vi "Put Multiple Files.vi"(3 "remote port (21)":u16=21, 4 "active (T)":bool=TRUE, 5 "password":string, 7 "user":string="anonymous", 8 "error in (no error)":errorcluster, 9 "Open Connection Timeout (ms)":dbl=5000.0, 10 "file specifications":T1(array[cluster]), 11 "host":string) -> (0 "error out":errorcluster, 2 "file errors":errorcluster[](array[cluster]))   [LabVIEW 2023]
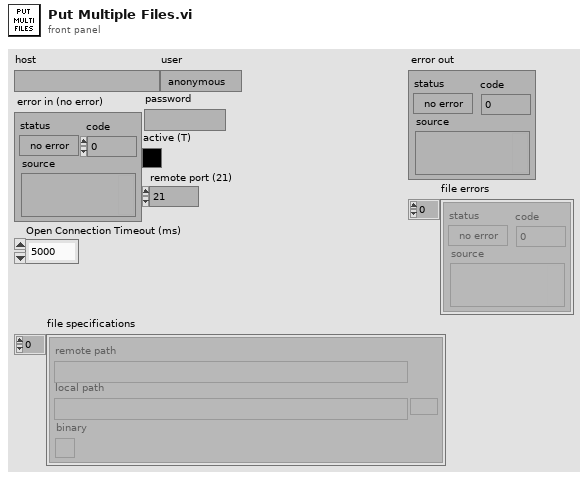
[diagram p1: front panel]
types:
  T1 = cluster{"remote path":string, "local path":path, "binary":bool}[]
  T2 = cluster{"remote path":string, "local path":path, "binary":bool, string}
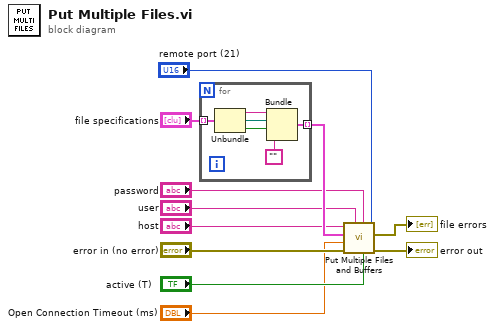
[diagram p0: block diagram]
diagram:
  n1 = for {
    tunnel: "file specifications" -> [w17] mode=indexing
    tunnel: [w12] -> w9 mode=indexing
    n2 = Unbundle(w17) -> ("remote path"=w16:string, "local path"=w15:path, "binary"=w14:bool)
    n3 = Bundle("remote path"=w16, "local path"=w15, "binary"=w14, "") -> (w12:T2)  [unwired: 1 out]
  }
  n4 = call "Put Multiple Files and Buffers.vi"("remote port (21)"="remote port (21)", "active (T)"="active (T)", "password"="password", "user"="user", "error in (no error)"="error in (no error)", "timeout ms (60000)"="Open Connection Timeout (ms)", "file specifications"=w9, "host"="host") -> ("error out"=→"error out":errorcluster, "file errors"=→"file errors":errorcluster[])  [unwired: 2 in]
